vi "Release Handle.vi"(8 "error in":errorcluster, 11 "session in":refnum<class "Session.lvclass">) -> (0 "error out":errorcluster, 3 "session out":refnum<class "Session.lvclass">)   [LabVIEW 2020, in "NI_SFTP.lvlib" / "Session.lvclass"]
uses:
  <vilib>/net/SFTP/Session/Session.lvclass
  <vilib>/net/SFTP/Session/Session.lvclass/Session.ctl
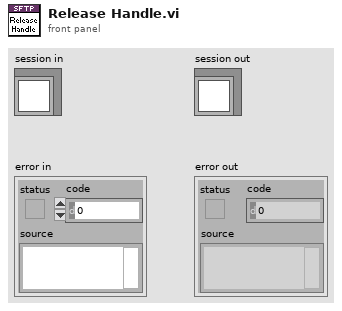
[diagram p1: front panel]
types:
  T1 = typedef "Semaphore RefNum" = refnum<k1>
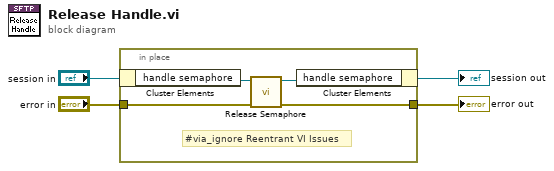
[diagram p0: block diagram]
diagram:
  n1 = in-place {
    in-place-border: "error in" -> [w6]
    in-place-border: [w5] -> w3
    # "#via_ignore Reentrant VI Issues"
    n2 = in-place-cluster #1("session in") -> ("handle semaphore"=w8:T1)
    n3 = call <vilib>:"Release Semaphore.vi"("error in (no error)"=w6, "semaphore"=w8) -> ("error out"=w5:errorcluster, "semaphore out"=w7:T1)  [unwired: 4 in]
    n4 = in-place-cluster #1("handle semaphore"=w7) -> (→"session out":refnum<class "Session.lvclass">)
  }
  "error out" <- w3
